vi "update_attrs.vi"(8 "error in (no error)":errorcluster, 10 "Nested Enqueuers Map":T1(c390), 11 "UDP_receiver in":refnum<class "UDP_receiver.lvclass">) -> (0 "error out":errorcluster, 3 "UDP_receiver out":refnum<class "UDP_receiver.lvclass">)   [LabVIEW 2025, in "UDP_receiver.lvlib" / "UDP_receiver.lvclass"]
uses:
  UDP_receiver.lvclass
  <vilib>/ActorFramework/Message Enqueuer/Message Enqueuer.lvclass
  UDP_receiver.lvclass/UDP_receiver.ctl
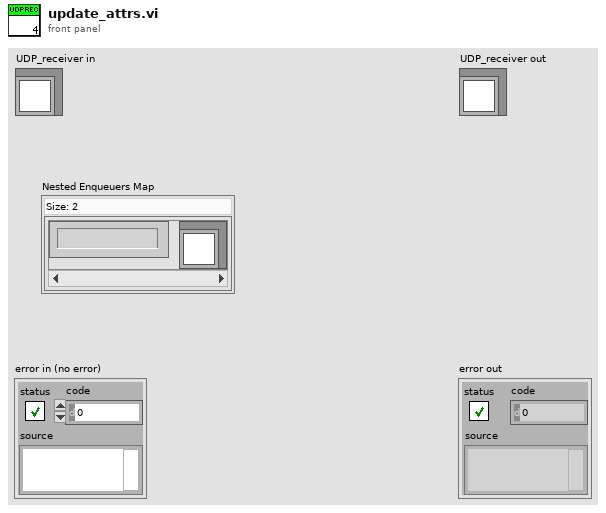
[diagram p1: front panel]
types:
  T1 = map{string, refnum<class "Message Enqueuer.lvclass">}
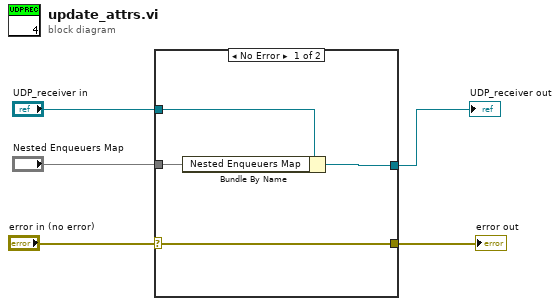
[diagram p0: block diagram]
diagram:
  n1 = case shown="No Error" "error in (no error)" {
    selector: "error in (no error)" -> [w6 w10]
    tunnel: "UDP_receiver in" -> [w9 w11]
    tunnel: [w8 w11] -> w4
    tunnel: "Nested Enqueuers Map" -> [w7 _]
    tunnel: [w6 w10] -> w1
    frame No Error {
      n2 = Bundle By Name(cluster=w9, "Nested Enqueuers Map"=w7) -> (w8:refnum<class "UDP_receiver.lvclass">)
    }
    frame Error {
    }
  }
  "error out" <- w1
  "UDP_receiver out" <- w4
